vi "Write ReadMode.vi"(8 "error in (no error)":errorcluster, 10 "ReadMode":T1(ring), 11 "Connection in":refnum<class "Connection.lvclass">) -> (0 "error out":errorcluster, 3 "Connection out":refnum<class "Connection.lvclass">)   [LabVIEW 2021, in "TcpServer.lvlib" / "Connection.lvclass"]
uses:
  Connection.lvclass
  Connection.lvclass/Connection.ctl
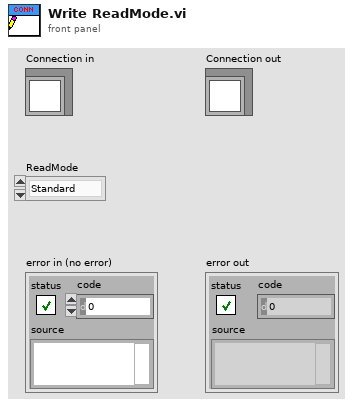
[diagram p1: front panel]
types:
  T1 = enum16{"Standard", "Buffered", "CRLF", "Immediate"}
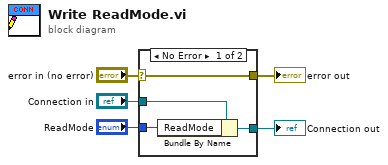
[diagram p0: block diagram]
diagram:
  n1 = case shown="No Error" "error in (no error)" {
    selector: "error in (no error)" -> [w9 w10]
    tunnel: [w9 w10] -> w4
    tunnel: [w7 w11] -> w2
    tunnel: "Connection in" -> [w8 w11]
    tunnel: "ReadMode" -> [w6 _]
    frame No Error {
      n2 = Bundle By Name(cluster=w8, "ReadMode"=w6) -> (w7:refnum<class "Connection.lvclass">)
    }
    frame Error {
    }
  }
  "error out" <- w4
  "Connection out" <- w2
